vi "SVL AC & DC Level (Frequency) (N Ch).vi"(0 "complex spectra":T7(array[cluster]) {"spectrum info"."x-axis units" items=["Time (s)"=0, "Frequency-CB (Hz)"=1, "Frequency-CPB (Hz)"=1248, "Frequency-Arbitrary (Hz)"=2357, "Quefrency (s)"=2, "Revolutions (rev)"=3, "Order"=4, "Speed (RPM)"=11, "Speed (rad/s)"=21, "Index"=65535]; "spectrum info"."weighting filter" items=["Linear", "A-weighting", "B-weighting", "C-weighting", "ITU-R 468-4", "Dolby", "CCITT", "C-message", "Wb", "Wc", "Wd", "We", "Wf", "Wh", "Wj", "Wk", "Wm", "AES17 20 kHz lowpass", "AES17 40 kHz lowpass", "AES17 20 kHz highpass", "AES17 40 kHz highpass"]; "spectrum info"."dB reference [EU]" format="%.2f"; "spectrum info"."engineering units" items=["custom..."=0, "V"=1, "A"=21, "C"=30, "pC"=31, "s"=32, "-"=29, "Pa"=2, "N"=20, "g"=3, "m/s^2"=4, "m/s"=5, "m"=6, "mm/s"=12, "mm"=13, "micron/s"=14, "micron"=15, "in/s^2"=7, "in/s"=8, "in"=9, "mil/s"=10, "mil"=11, "rad/s^2"=16, "rad/s"=17, "rad"=18, "deg/s^2"=26, "deg/s"=27, "deg"=28, "RPM"=22, "cycle/s^2"=23, "Hz"=24, "cycle"=25, "strain"=19]; "spectrum info"."spectral info"."window" items=["None "=0, "Hanning"=1, "Hamming"=2, "Blackman-Harris"=3, "Exact Blackman"=4, "Blackman"=5, "Flat Top"=6, "4 Term B-Harris "=7, "7 Term B-Harris"=8, "Low Sidelobe"=9, "Force - Exponential"=10, "Gaussian"=62]; "complex spectrum response"."complex spectrum" format="%.2f"; "complex spectrum response"."df" format="%.2f"; "complex spectrum response"."f0" format="%.2f"}, 5 "error in (no error)":errorcluster) -> (12 "unit labels":string[](array[string]), 14 "AC complex spectra":T7(array[cluster]) {"spectrum info"."x-axis units" items=["Time (s)"=0, "Frequency-CB (Hz)"=1, "Frequency-CPB (Hz)"=1248, "Frequency-Arbitrary (Hz)"=2357, "Quefrency (s)"=2, "Revolutions (rev)"=3, "Order"=4, "Speed (RPM)"=11, "Speed (rad/s)"=21, "Index"=65535]; "spectrum info"."weighting filter" items=["Linear", "A-weighting", "B-weighting", "C-weighting", "ITU-R 468-4", "Dolby", "CCITT", "C-message", "Wb", "Wc", "Wd", "We", "Wf", "Wh", "Wj", "Wk", "Wm", "AES17 20 kHz lowpass", "AES17 40 kHz lowpass", "AES17 20 kHz highpass", "AES17 40 kHz highpass"]; "spectrum info"."dB reference [EU]" format="%.2f"; "spectrum info"."engineering units" items=["custom..."=0, "V"=1, "A"=21, "C"=30, "pC"=31, "s"=32, "-"=29, "Pa"=2, "N"=20, "g"=3, "m/s^2"=4, "m/s"=5, "m"=6, "mm/s"=12, "mm"=13, "micron/s"=14, "micron"=15, "in/s^2"=7, "in/s"=8, "in"=9, "mil/s"=10, "mil"=11, "rad/s^2"=16, "rad/s"=17, "rad"=18, "deg/s^2"=26, "deg/s"=27, "deg"=28, "RPM"=22, "cycle/s^2"=23, "Hz"=24, "cycle"=25, "strain"=19]; "spectrum info"."spectral info"."window" items=["None "=0, "Hanning"=1, "Hamming"=2, "Blackman-Harris"=3, "Exact Blackman"=4, "Blackman"=5, "Flat Top"=6, "4 Term B-Harris "=7, "7 Term B-Harris"=8, "Low Sidelobe"=9, "Force - Exponential"=10, "Gaussian"=62]; "complex spectrum response"."complex spectrum" format="%.2f"; "complex spectrum response"."df" format="%.2f"; "complex spectrum response"."f0" format="%.2f"}, 15 "AC levels [EU rms]":dbl[](array[numeric]) format="%.8f", 16 "DC complex spectra":T7(array[cluster]) {"spectrum info"."x-axis units" items=["Time (s)"=0, "Frequency-CB (Hz)"=1, "Frequency-CPB (Hz)"=1248, "Frequency-Arbitrary (Hz)"=2357, "Quefrency (s)"=2, "Revolutions (rev)"=3, "Order"=4, "Speed (RPM)"=11, "Speed (rad/s)"=21, "Index"=65535]; "spectrum info"."weighting filter" items=["Linear", "A-weighting", "B-weighting", "C-weighting", "ITU-R 468-4", "Dolby", "CCITT", "C-message", "Wb", "Wc", "Wd", "We", "Wf", "Wh", "Wj", "Wk", "Wm", "AES17 20 kHz lowpass", "AES17 40 kHz lowpass", "AES17 20 kHz highpass", "AES17 40 kHz highpass"]; "spectrum info"."dB reference [EU]" format="%.2f"; "spectrum info"."engineering units" items=["custom..."=0, "V"=1, "A"=21, "C"=30, "pC"=31, "s"=32, "-"=29, "Pa"=2, "N"=20, "g"=3, "m/s^2"=4, "m/s"=5, "m"=6, "mm/s"=12, "mm"=13, "micron/s"=14, "micron"=15, "in/s^2"=7, "in/s"=8, "in"=9, "mil/s"=10, "mil"=11, "rad/s^2"=16, "rad/s"=17, "rad"=18, "deg/s^2"=26, "deg/s"=27, "deg"=28, "RPM"=22, "cycle/s^2"=23, "Hz"=24, "cycle"=25, "strain"=19]; "spectrum info"."spectral info"."window" items=["None "=0, "Hanning"=1, "Hamming"=2, "Blackman-Harris"=3, "Exact Blackman"=4, "Blackman"=5, "Flat Top"=6, "4 Term B-Harris "=7, "7 Term B-Harris"=8, "Low Sidelobe"=9, "Force - Exponential"=10, "Gaussian"=62]; "complex spectrum response"."complex spectrum" format="%.2f"; "complex spectrum response"."df" format="%.2f"; "complex spectrum response"."f0" format="%.2f"}, 17 "DC levels [EU]":dbl[](array[numeric]) format="%0.2f", 19 "error out":errorcluster)   [LabVIEW 2017]
doc: "Computes the AC level and DC level of a signal. Wire data to the <B>scaled signal [EU]</B> input to determine the polymorphic instance to use or manually select the instance."
uses:
  <vilib>/addons/_NISVFA/_Shared subVIs/Controls/svc_Spectrum Info.ctl
  <vilib>/addons/_NISVFA/_Shared subVIs/Controls/svc_X-Axis Units.ctl
  <vilib>/addons/_NISVFA/_Shared subVIs/Controls/svc_Spectrum Type.ctl
  <vilib>/addons/_NISVFA/_Shared subVIs/Controls/svc_Engineering Units Text Ring.ctl
  <vilib>/addons/_NISVFA/_Shared subVIs/Controls/svc_Weighting Filter Text Ring.ctl
  <vilib>/addons/_NISVFA/_Shared subVIs/Controls/svc_Complimentary Spectrum Units.ctl
  <vilib>/Analysis/2dsp.llb/Real FFT.vi
  <vilib>/Analysis/baseanly.llb/Mean (DBL).vi
  <vilib>/Analysis/4window.llb/Force Window.vi
  <vilib>/Analysis/4window.llb/Force Window (DBL).vi
  <vilib>/Analysis/4window.llb/Exponential Window.vi
  <vilib>/Analysis/4window.llb/Exponential Window (DBL).vi
  <vilib>/addons/_NISVFA/_Shared subVIs/Common/svc_Get Weighting Enum and Labels.vi
  <vilib>/addons/_NISVFA/_Shared subVIs/Common/svc_Unit Label Lexical Class.vi
  <vilib>/addons/_NISVFA/_Shared subVIs/Common/svc_Engineering Units to Unit Label.vi
  <vilib>/addons/_NISVFA/_Shared subVIs/Common/svc_Format Value (DBL).vi
  <vilib>/Utility/error.llb/Error Cluster From Error Code.vi
  <vilib>/Analysis/0measdsp.llb/Scaled Time Domain Window.vi
  <vilib>/Analysis/0measdsp.llb/Scaled Time Domain Window (DBL).vi
  <vilib>/addons/_NISVFA/_Spectrum Processing/subVIs/svfa_Spectrum Info Window to windowTd Type Def.vi
  <vilib>/Analysis/NI_AALPro.lvlib
  <vilib>/Analysis/NI_AALBase.lvlib
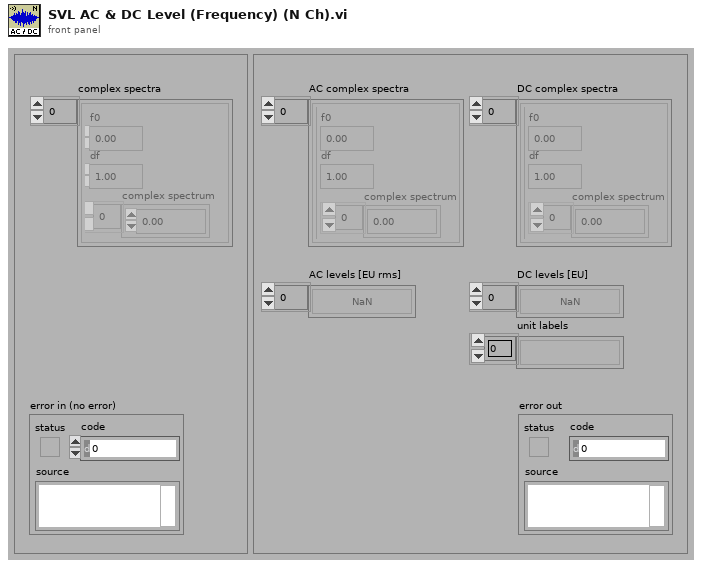
[diagram p1: front panel]
types:
  T1 = typedef "svc_Spectrum Info.ctl" = cluster{"channel name":string, "description":string, "x-axis units":T2, "spectral info":cluster{"spectrum type":T3, "linear/dB":enum16{"linear", "dB"}, "window":u16, "window size":i32, "FFT size":i32}, "engineering units":T4, "custom label":string, "dB reference [EU]":dbl, "peak units":enum16{"rms", "peak", "peak-peak"}, "weighting filter":T5, "spectral density?":bool, "unit label":string, "spectrum skewed?":bool, "complimentary spectrum units":T6}
  T2 = typedef "svc_X-Axis Units.ctl" = u16
  T3 = typedef "svc_Spectrum Type.ctl" = enum16{"FFT Spectrum [complex]", "Amplitude [Magnitude]", "Power [Magnitude^2]", "Cross Spectrum [complex]", "Frequency Response [Complex]"}
  T4 = typedef "svc_Engineering Units Text Ring.ctl" = u16
  T5 = typedef "svc_Weighting Filter Text Ring.ctl" = u16
  T6 = typedef "svc_Complimentary Spectrum Units.ctl" = enum16{"none", "radians", "degrees", "cycles", "imaginary"}
  T7 = cluster{"complex spectrum response":cluster{"f0":dbl, "df":dbl, "complex spectrum":cdb[]}, "spectrum info":T1}[]
  T8 = cluster{"complex spectrum response":cluster{"f0":dbl, "df":dbl, "complex spectrum":cdb[]}, "spectrum info":T1}
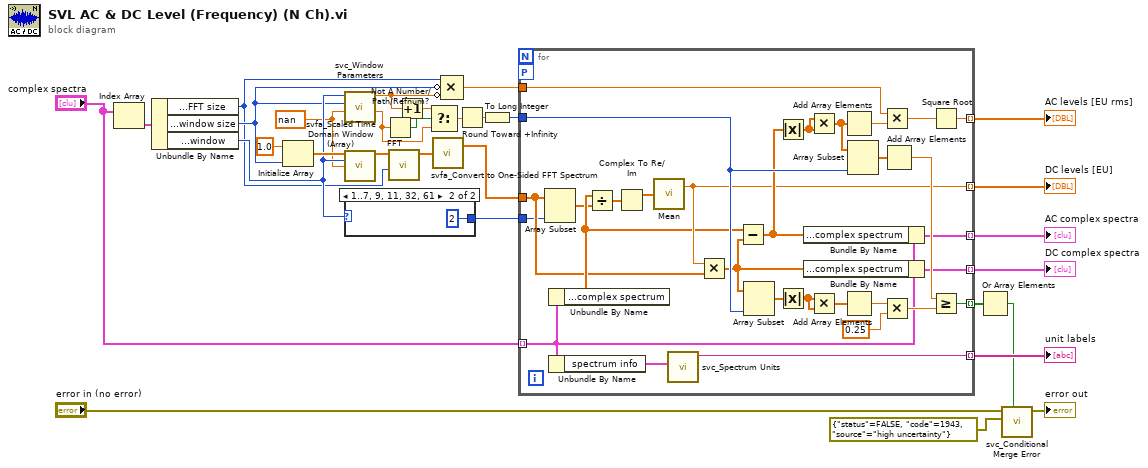
[diagram p0: block diagram]
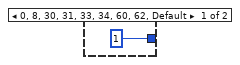
[diagram p2: hidden frame]
diagram:
  w6 = nan ("window parameter")
  n1 = Index Array(array="complex spectra") -> (element=w9:T8)  [unwired: 1 in]
  n2 = Unbundle By Name(w9) -> ("spectrum info.spectral info.FFT size"=w1:i32, "spectrum info.spectral info.window size"=w11:i32, "spectrum info.spectral info.window"=w13:u16)
  n3 = Initialize Array(1.0 ("element"), w11) -> (w17:dbl[])
  n4 = call <vilib>:"svc_Window Parameters.vi"("standard deviation"=w6, "window size"=w11, "window"=w13) -> ("6dB BW"=w27:dbl, "ENBW"=w29:dbl)  [unwired: 5 in, 2 out]
  n5 = call <vilib>:"svfa_Scaled Time Domain Window (Array).vi"("input signal"=w17, "window"=w13, "window parameter"=w6) -> ("windowed signal"=w18:dbl[])  [unwired: 7 in, 5 out]
  n6 = case shown="1..7, 9, 11, 32, 61" w13 {
    tunnel: [1 ("length") 2 ("length")] -> w7
    frame 0, 8, 30, 31, 33, 34, 60, 62, Default {
    }
    frame 1..7, 9, 11, 32, 61 {
    }
  }
  n7 = Not A Number/Path/Refnum?(number/path/refnum=w27) -> (NaN/Path/Refnum?=w26:bool)
  n8 = call-poly <vilib>:"FFT.vi"("FFT size"=w1, "X"=w18) -> ("FFT {X}"=w16:cdb[])  [unwired: 8 in, 1 out]
  n9 = Increment(x=w29) -> (x+1=w28:dbl)
  n10 = Select(t=w28, s=w26, f=w27) -> (s? t:f=w30:dbl)
  n11 = call <vilib>:"svfa_Convert to One-Sided FFT Spectrum.vi"("two-sided FFT spectrum"=w16) -> ("one-sided FFT spectrum"=w8:cdb[])  [unwired: 1 out]
  n12 = Compound Arithmetic op=MULTIPLY(w1, invert w11, invert w29) -> (w12:dbl)
  n13 = Round Toward +Infinity(x=w30) -> (ceil(x): smallest int >= x=w23:dbl)
  n14 = To Long Integer(number=w23) -> (32bit integer=w24:i32)
  n15 = for {
    tunnel: [w59] -> w25 mode=indexing
    tunnel: w24 -> [w58]
    tunnel: [w49] -> w22 mode=indexing
    tunnel: [w47] -> w21 mode=indexing
    tunnel: [w46] -> w20 mode=indexing
    tunnel: [w45] -> w19 mode=indexing
    tunnel: [w42] -> w14 mode=indexing
    tunnel: w12 -> [w40]
    tunnel: "complex spectra" -> [w36] mode=indexing
    tunnel: w8 -> [w35]
    tunnel: w7 -> [w34]
    workers-P: _ -> [_]
    n16 = Array Subset(array=w35, length=w34) -> (w33:cdb[])  [unwired: 1 in]
    n17 = Unbundle By Name(w36) -> ("complex spectrum response.complex spectrum"=w38:cdb[])
    n18 = Unbundle By Name(w36) -> ("spectrum info"=w37:T1)
    n19 = Divide(x=w38, y=w33) -> (x/y=w43:cdb[])
    n20 = Complex To Re/Im(x + iy=w43) -> (x=w44:dbl[])  [unwired: 1 out]
    n21 = call-poly <vilib>:"Mean.vi"("X"=w44) -> ("mean"=w45:dbl)  [unwired: 1 out]
    n22 = call <vilib>:"svc_Spectrum Units.vi"("spectrum info in"=w37) -> ("unit label"=w42:string)  [unwired: 3 in, 3 out]
    n23 = Multiply(x=w45, y=w35) -> (x*y=w51:cdb[])
    n24 = Subtract(x=w38, y=w51) -> (x-y=w48:cdb[])
    n25 = Array Subset(array=w51, length=w58) -> (w54:cdb[])  [unwired: 1 in]
    n26 = Absolute Value(x=w48) -> (abs(x)=w52:dbl[])
    n27 = Absolute Value(x=w54) -> (abs(x)=w60:dbl[])
    n28 = Bundle By Name(cluster=w36, "complex spectrum response.complex spectrum"=w48) -> (w47:T8)
    n29 = Bundle By Name(cluster=w36, "complex spectrum response.complex spectrum"=w51) -> (w46:T8)
    n30 = Multiply(x=w52, y=w52) -> (x*y=w53:dbl[])
    n31 = Multiply(x=w60, y=w60) -> (x*y=w50:dbl[])
    n32 = Add Array Elements(numeric array=w53) -> (sum=w41:dbl)
    n33 = Add Array Elements(numeric array=w50) -> (sum=w57:dbl)
    n34 = Array Subset(array=w53, length=w58) -> (w55:dbl[])  [unwired: 1 in]
    n35 = Multiply(x=w40, y=w41) -> (x*y=w39:dbl)
    n36 = Multiply(x=w57, y=0.25) -> (x*y=w61:dbl)
    n37 = Add Array Elements(numeric array=w55) -> (sum=w56:dbl)
    n38 = Square Root(x=w39) -> (sqrt(x)=w49:dbl)
    n39 = Greater Or Equal?(x=w56, y=w61) -> (x >= y?=w59:bool)
  }
  "AC levels [EU rms]" <- w22
  "AC complex spectra" <- w21
  "DC complex spectra" <- w20
  "DC levels [EU]" <- w19
  "unit labels" <- w14
  n40 = Or Array Elements(Boolean array=w25) -> (logical OR=w4:bool)
  n41 = call <vilib>:"svc_Conditional Merge Error.vi"("merge"=w4, "new error"=errorcluster {"status"=FALSE, "code"=1943, "source"="high uncertainty"} ("error in 2 (no error)"), "error in (no error)"="error in (no error)") -> ("error out"=→"error out":errorcluster)  [unwired: 8 in]
